vi "caiquan1 radom.vi"(8 "错误输入（无错误）":errorcluster, 10 "挑战者输入":u16, 11 ".NET引用句柄输入":refnum<k24>) -> (0 "错误输出":errorcluster, 1 "IsEmpty":bool, 2 "挑战者输出":u16, 3 ".NET引用句柄输出":refnum<k24>)   [LabVIEW 2016]
uses:
  D:/Program Files (x86)/National Instruments/LabVIEW 2016/vi.lib/MakerHub/Leap/Private/Libs/LeapCSharp.NET3.5.dll
  Program Files (x86)/National Instruments/LabVIEW 2016/vi.lib/MakerHub/Leap/Private/Libs/LeapCSharp.NET3.5.dll
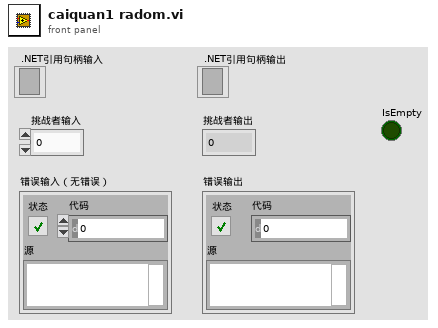
[diagram p1: front panel]
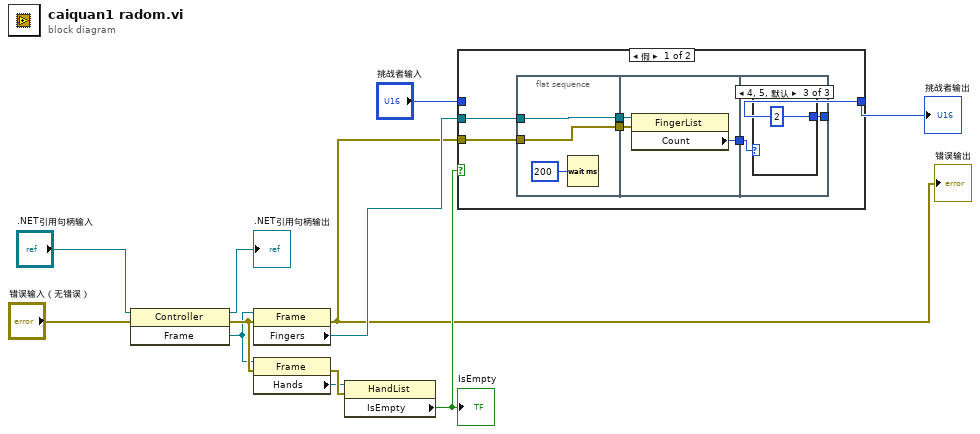
[diagram p0: block diagram]
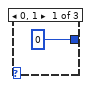
[diagram p2: hidden frame]
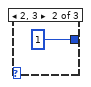
[diagram p3: hidden frame]
diagram:
  n1 = invoke class="Controller" method="Frame"(reference=".NET引用句柄输入", error in="错误输入（无错误）") -> (reference out=→".NET引用句柄输出":refnum<k24>, error out=w8:errorcluster, "Frame"=w7:refnum<k24>)  [unwired: 1 in]
  n2 = property class="Frame"(reference=w7, error in=w8) -> (error out=w1:errorcluster, "Fingers"=w2:refnum<k24>)  [unwired: 1 out]
  "错误输出" <- w1
  n3 = property class="Frame"(reference=w7, error in=w8) -> (error out=w10:errorcluster, "Hands"=w9:refnum<k24>)  [unwired: 1 out]
  n4 = property class="HandList"(reference=w9, error in=w10) -> ("IsEmpty"=w3:bool)  [unwired: 2 out]
  "IsEmpty" <- w3
  n5 = case shown="假" w3 {
    tunnel: [w18 w30] -> w12
    tunnel: "挑战者输入" -> [_ w30]
    tunnel: w2 -> [w16 _]
    tunnel: w1 -> [w15 _]
    frame False {
      n6 = flat-sequence {
        tunnel: [w20] -> w17
        tunnel: w16 -> [w20]
        tunnel: w15 -> [w19]
        tunnel: [w19] -> w14
        tunnel: w17 -> [w24]
        tunnel: w14 -> [w23]
        tunnel: [w22] -> w13
        tunnel: [w26] -> w18
        tunnel: w13 -> [w25]
        frame #0 {
          n7 = Wait (ms)(milliseconds to wait=u32 200 ("等待时间（毫秒）")) -> ()  [unwired: 1 out]
        }
        frame #1 {
          n8 = property class="FingerList"(reference=w24, error in=w23) -> ("Count"=w22:i32)  [unwired: 2 out]
        }
        frame #2 {
          n9 = case shown="4, 5, 默认" w25 {
            tunnel: [u16 0 ("挑战者") u16 1 ("挑战者") u16 2 ("挑战者")] -> w26
            frame 0, 1 {
            }
            frame 2, 3 {
            }
            frame 4, 5, Default {
            }
          }
        }
      }
    }
    frame True {
    }
  }
  "挑战者输出" <- w12
